vi "UI - Configuration.vi"() -> ()   [LabVIEW 2020, in "Logger.lvlib" / "Configuration.lvclass"]
doc: "Module UI that appears in the Configuration UI.\n____\nPeloton Config 2.0.0.9\nCopyright (c) 2024, Peloton"
uses:
  Configuration.lvclass
  <vilib>/Peloton/Peloton Config/DCFG Framework/Init UI Params--cluster.ctl
  <vilib>/Peloton/Peloton Config/DCFG Framework/Configuration_class/Configuration.lvclass
  <vilib>/Peloton/Peloton Config/DCFG Framework/Stop Argument--cluster.ctl
  <vilib>/Peloton/Peloton Config/DCFG Framework/Send Config to Page Argument--cluster.ctl
  <vilib>/Peloton/Peloton Config/DCFG Framework/Send Stop to Page Argument--cluster.ctl
  C:/Program Files (x86)/National Instruments/LabVIEW 2020/vi.lib/Peloton/Peloton Config/DCFG Framework/Configuration_class/Configuration.lvclass
  <vilib>/Peloton/Peloton Config/DCFG Framework/Configuration_class/Configuration.lvclass/Configuration.ctl
  Configuration--cluster.ctl
  Configuration.lvclass/Configuration.ctl
  Set Configuration.vi
  Get Configuration.vi
  <vilib>/Peloton/Peloton Config/DCFG Framework/Configuration_class/Get Name.vi
  <vilib>/Peloton/Peloton Config/DCFG Framework/Peloton_lib_DCFG Framework.lvlib
panel:
  in  "File Path":path
  in  "Init UI Params":T1
  # "Define the Default Configuration UI here."
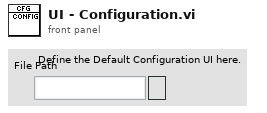
[diagram p1: front panel]
types:
  T1 = typedef "Peloton_lib_DCFG Framework.lvlib/Init UI Params--cluster.ctl" = cluster{"Initial Config":refnum<class "Configuration.lvclass">, "Stop CFG Module":refnum<user-event>, "Send Config to Page":refnum<user-event>, "Send Stop to Page":refnum<user-event>, "Reset Page Defaults":refnum<user-event>}
  T2 = enum32{"Invalid", "Standard", "Closed", "Hidden", "Minimized", "Maximized"}
  T3 = typedef "Logger.lvlib/Configuration.lvclass/Configuration--cluster.ctl" = cluster{"File Path":path}
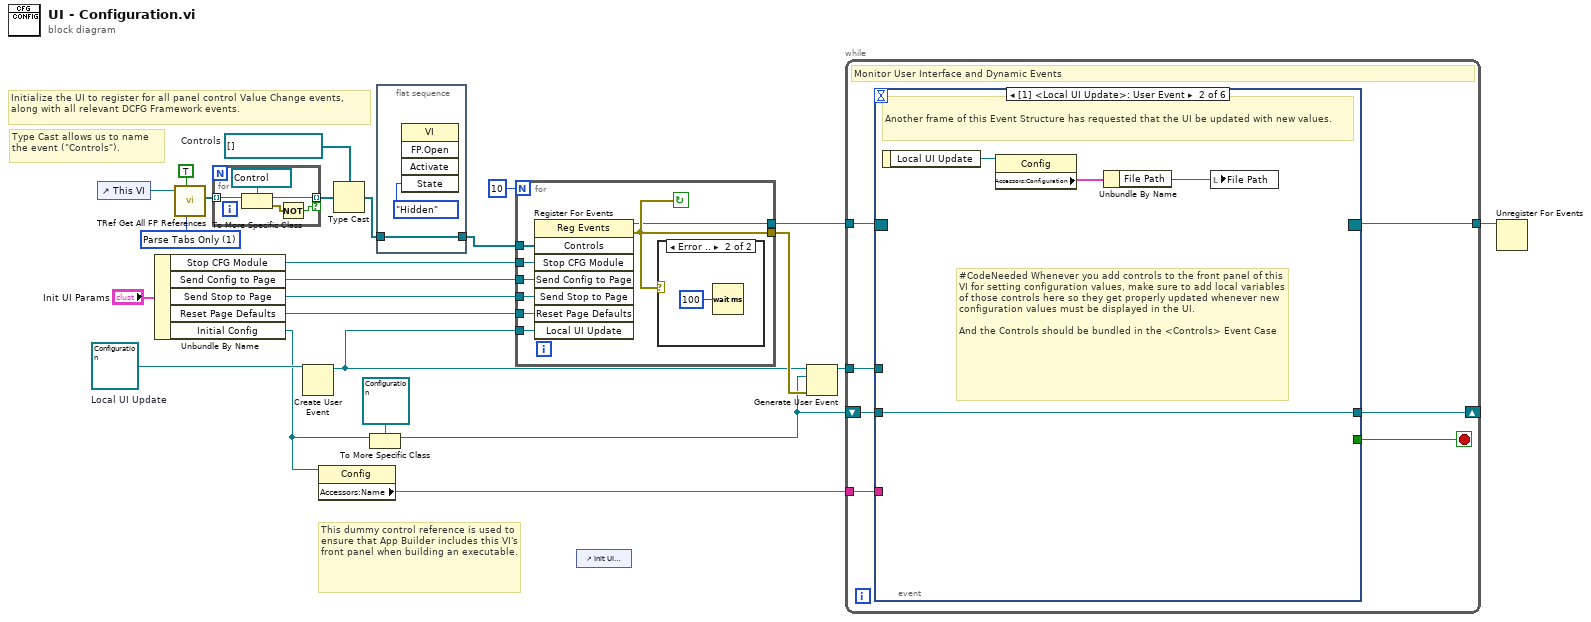
[diagram p0: block diagram]
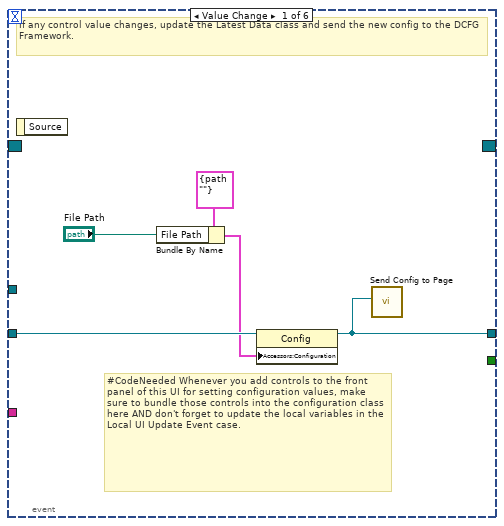
[diagram p3: hidden frame]
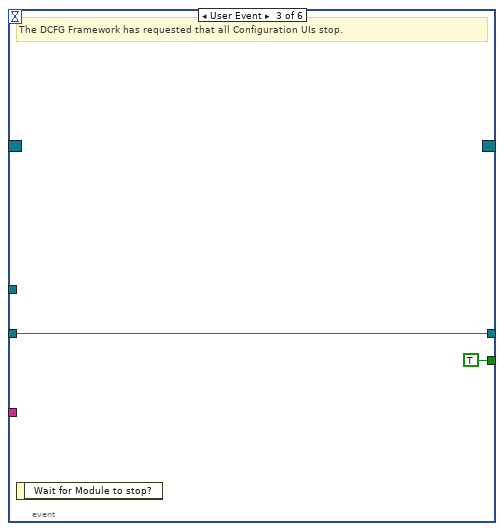
[diagram p4: hidden frame]
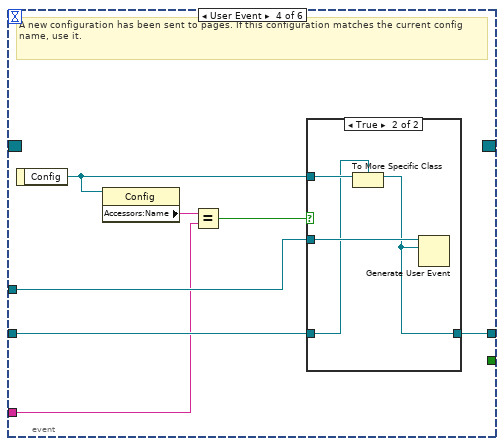
[diagram p5: hidden frame]
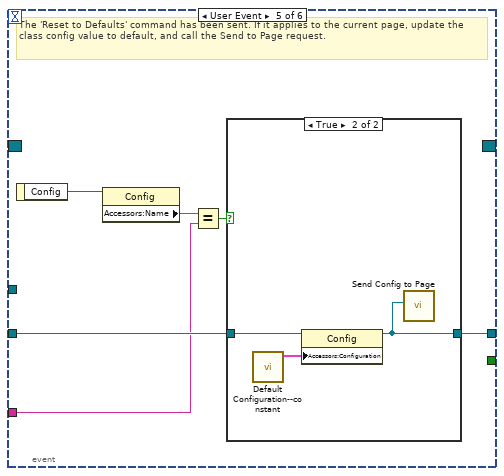
[diagram p7: hidden frame]
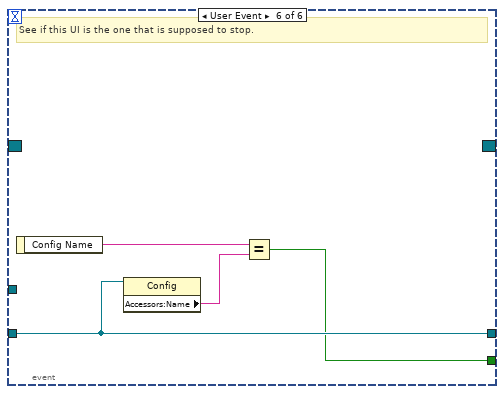
[diagram p9: hidden frame]
diagram:
  w6 = refnum<vi>[] []  # Controls
  w11 = u16 1 items=["Parse All", "Parse Tabs Only"] ("Parsing Rule")
  w21 = refnum<class "Configuration.lvclass"> refnum  # Local UI Update
  # "Type Cast allows us to name the event (\"Controls\")."
  # "Initialize the UI to register for all panel control Value Change events, along with all relevant DCFG Framework events."
  # "This dummy control reference is used to ensure that App Builder includes this VI's front panel when building an executable."
  n1 = control-ref of="This VI"() -> (w1:refnum<vi>)
  n2 = Unbundle By Name("Init UI Params") -> ("Stop CFG Module"=w18:refnum<user-event>, "Send Config to Page"=w17:refnum<user-event>, "Send Stop to Page"=w16:refnum<user-event>, "Reset Page Defaults"=w15:refnum<user-event>, "Initial Config"=w8:refnum<class "Configuration.lvclass">)
  n3 = call <vilib>:"TRef Get All FP References.vi"("Parsing Rule"=w11, "Ignore Decorations?"=TRUE, "VI Refnum"=w1) -> ("All FP Objects"=w12:refnum<vi>[])  [unwired: 4 in, 4 out]
  n4 = for {
    tunnel: w12 -> [w28] mode=indexing
    tunnel: [w27] -> w5 mode=indexing if=w25
    n5 = To More Specific Class(target class=refnum<vi> refnum ("Controls"), reference=w28) -> (specific class reference=w27:refnum<vi>, error out=w29:errorcluster)  [unwired: 1 in]
    n6 = Not(x=w29) -> (.not. x?=w25:bool)
  }
  n7 = Create User Event(user event datatype=w21) -> (user event=w14:refnum<user-event>)  [unwired: 1 in, 1 out]
  n8 = property class="Config"(reference=w8) -> ("Accessors:Name"=w7:string)  [unwired: 1 in, 2 out]
  n9 = Type Cast(type=w6, x=w5) -> (*(type *) &x=w4:refnum<vi>[])
  n10 = To More Specific Class(target class=refnum<class "Configuration.lvclass"> refnum ("Sample Module 1.lvlib:Config"), reference=w8) -> (specific class reference=w10:refnum<class "Configuration.lvclass">)  [unwired: 1 in, 1 out]
  n11 = flat-sequence {
    tunnel: w4 -> [w31]
    tunnel: [w31] -> w3
    frame #0 {
      n12 = invoke on="Invoke Node" class="VI" method="FP.Open"("State"=T2."Hidden") -> ()  [unwired: 4 in, 5 out]
    }
  }
  n13 = for {
    N: 10 -> [_]
    tunnel: [w38] -> w23
    tunnel: [w39] -> w24
    tunnel: w18 -> [w37]
    tunnel: w17 -> [w36]
    tunnel: w16 -> [w35]
    tunnel: w15 -> [w34]
    tunnel: w14 -> [w33]
    tunnel: w3 -> [w32]
    stop <- w39 continue-if-true
    n14 = register-events(w32, w37, w36, w35, w34, w33) -> (reference out=w38:refnum<event-registration>, error out=w39:errorcluster)  [unwired: 2 in]
    n15 = case shown="Error .." w39 {
      frame No Error {
      }
      frame Error {
        n16 = Wait (ms)(milliseconds to wait=u32 100) -> ()  [unwired: 1 out]
      }
    }
  }
  n17 = control-ref of="Init UI Params"() -> ()  [unwired: 1 out]
  n18 = Generate User Event(user event=w14, event data cluster=w10, error in=w24) -> (user event out=w20:refnum<user-event>)  [unwired: 1 in, 1 out]
  n19 = while {
    tunnel: w23 -> [w47]
    tunnel: [w46] -> w22
    shift-right: [w42] -> _
    shift-left: w10 -> [w45]
    tunnel: w20 -> [w43]
    tunnel: w7 -> [w41]
    stop <- w44 stop-if-true
    # "Monitor User Interface and Dynamic Events"
    n20 = event shown="[1] <Local UI Update>: User Event" {
      selector: w47 -> [_ _ _ _ _ _]
      dyn-events: [_ _ _ _ _ _] -> w46
      timeout: _ -> [_ _ _ _ _ _]
      tunnel: w45 -> [w51 w56 w58 w63 w75 w84]
      tunnel: [w50 w56 w58 w64 w76 w84] -> w42
      tunnel: [_ _ TRUE ("Addressed to this instance?") _ _ w81] -> w44
      tunnel: w43 -> [_ _ _ w65 _ _]
      tunnel: w41 -> [_ _ _ w60 w72 _]
      event Value Change {
        # "#CodeNeeded Whenever you add controls to the front panel of this UI for setting configuration values, make sure to bundle those controls into the configuration class here AND don't forget to update the local variables in the Local UI Update Event case."
        # "If any control value changes, update the Latest Data class and send the new config to the DCFG Framework."
        n21 = event-data() -> ()  [unwired: 1 in, 1 out]
        n22 = Bundle By Name(cluster=T3 {"File Path"=path ""} ("Configuration"), "File Path"="File Path") -> (w49:T3)
        n23 = property class="Config"(reference=w51, "Accessors:Configuration"=w49) -> (reference out=w50:refnum<class "Configuration.lvclass">)  [unwired: 1 in, 1 out]
        n24 = call <vilib>:"Send Config to Page.vi"("Config"=w50) -> ()  [unwired: 10 in, 1 out]
      }
      event User Event {
        # "#CodeNeeded Whenever you add controls to the front panel of this VI for setting configuration values, make sure to add local variables of those controls here so they get properly updated whenever new configuration values must be displayed in the UI.\n\nAnd the Controls should be bundled in the <Controls> Event Case"
        # "Another frame of this Event Structure has requested that the UI be updated with new values."
        n25 = event-data() -> ("Local UI Update"=w55:refnum<class "Configuration.lvclass">)  [unwired: 1 in]
        n26 = property class="Config"(reference=w55) -> ("Accessors:Configuration"=w54:T3)  [unwired: 1 in, 2 out]
        n27 = Unbundle By Name(w54) -> ("File Path"=w53:path)
        n28 = local write "File Path"(w53) -> ()
      }
      event User Event {
        # "The DCFG Framework has requested that all Configuration UIs stop."
        n29 = event-data() -> ()  [unwired: 1 in, 1 out]
      }
      event User Event {
        # "A new configuration has been sent to pages. If this configuration matches the current config name, use it."
        n30 = event-data() -> ("Config"=w62:refnum<class "Configuration.lvclass">)  [unwired: 1 in]
        n31 = property class="Config"(reference=w62) -> ("Accessors:Name"=w61:string)  [unwired: 1 in, 2 out]
        n32 = Equal?(x=w61, y=w60) -> (x = y?=w59:bool)
        n33 = case shown="True" w59 {
          tunnel: w65 -> [_ w70]
          tunnel: w63 -> [w66 w67]
          tunnel: [w66 w69] -> w64
          tunnel: w62 -> [_ w68]
          frame False {
          }
          frame True {
            n34 = To More Specific Class(target class=w67, reference=w68) -> (specific class reference=w69:refnum<class "Configuration.lvclass">)  [unwired: 1 in, 1 out]
            n35 = Generate User Event(user event=w70, event data cluster=w69) -> ()  [unwired: 2 in, 2 out]
          }
        }
      }
      event User Event {
        # "The 'Reset to Defaults' command has been sent. If it applies to the current page, update the class config value to default, and call the Send to Page request."
        n36 = event-data() -> ("Config"=w74:refnum<class "Configuration.lvclass">)  [unwired: 1 in]
        n37 = property class="Config"(reference=w74) -> ("Accessors:Name"=w73:string)  [unwired: 1 in, 2 out]
        n38 = Equal?(x=w73, y=w72) -> (x = y?=w71:bool)
        n39 = case shown="True" w71 {
          tunnel: w75 -> [w77 w80]
          tunnel: [w77 w78] -> w76
          frame False {
          }
          frame True {
            n40 = call "Default Configuration--constant.vi"() -> ("Default Configuration"=w79:T3)  [unwired: 11 in]
            n41 = property class="Config"(reference=w80, "Accessors:Configuration"=w79) -> (reference out=w78:refnum<class "Configuration.lvclass">)  [unwired: 1 in, 1 out]
            n42 = call <vilib>:"Send Config to Page.vi"("Config"=w78) -> ()  [unwired: 10 in, 1 out]
          }
        }
      }
      event User Event {
        # "See if this UI is the one that is supposed to stop."
        n43 = event-data() -> ("Config Name"=w83:string)  [unwired: 1 in]
        n44 = property class="Config"(reference=w84) -> ("Accessors:Name"=w82:string)  [unwired: 1 in, 2 out]
        n45 = Equal?(x=w83, y=w82) -> (x = y?=w81:bool)
      }
    }
  }
  n46 = Unregister For Events(event registration refnum=w22) -> ()  [unwired: 1 in, 1 out]
